vi "ConexionSerial_Clase3.vi"() -> ()   [LabVIEW 2017]
uses:
  <vilib>/Instr/_visa.llb/VISA Configure Serial Port (Instr).vi
panel:
  out "x+/-y":i8
  in  "stop":bool
  out "read buffer":string
  in  "VISA resource name":refnum<visa-resource-name>
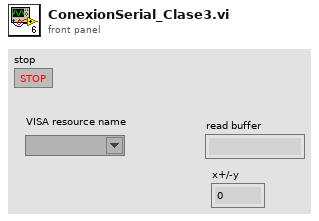
[diagram p1: front panel]
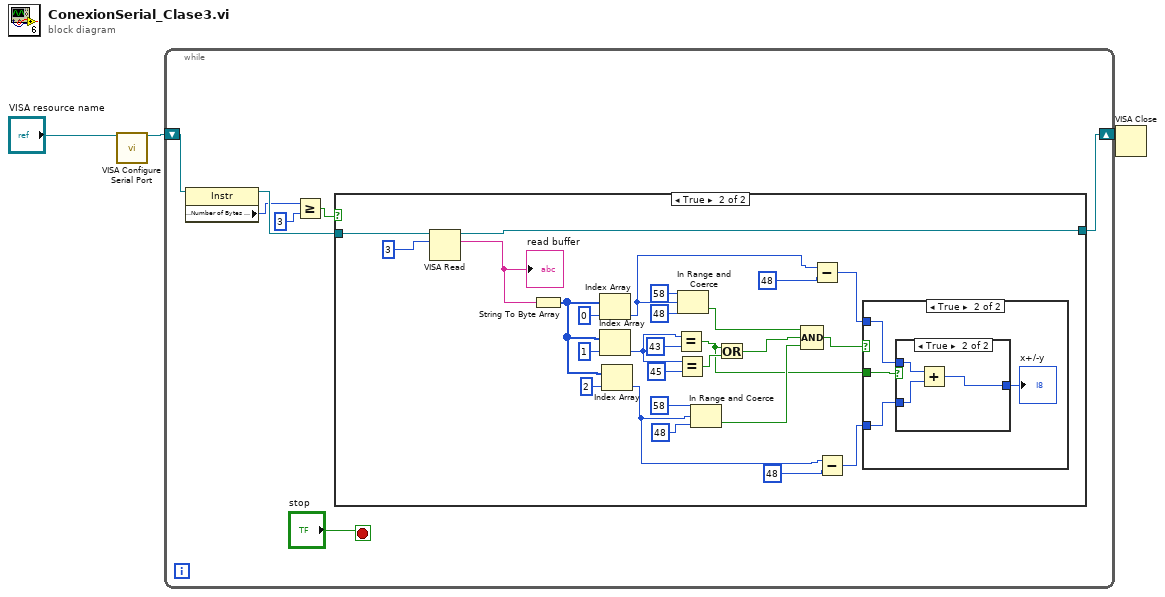
[diagram p0: block diagram]
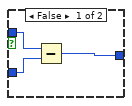
[diagram p4: hidden frame]
diagram:
  n1 = call-poly "VISA Configure Serial Port"("VISA resource name"="VISA resource name") -> ("VISA resource name out"=w2:refnum<visa-resource-name>)  [unwired: 13 in, 1 out]
  n2 = while {
    shift-right: [w10] -> w1
    shift-left: w2 -> [w8]
    stop <- "stop" stop-if-true
    n3 = property class="Instr"(reference=w8) -> (reference out=w7:refnum<visa-resource-name>, "Serial Settings:Number of Bytes at Serial Port"=w4:u32)  [unwired: 1 in, 1 out]
    n4 = Greater Or Equal?(x=w4, y=u32 3 ("x")) -> (x >= y?=w6:bool)
    n5 = case shown="True" w6 {
      tunnel: w7 -> [w11 w38]
      tunnel: [w11 w36] -> w10
      frame False {
      }
      frame True {
        n6 = VISA Read(VISA resource name=w38, byte count=u32 3) -> (VISA resource name out=w36:refnum<visa-resource-name>, read buffer=w35:string)  [unwired: 1 in, 2 out]
        "read buffer" <- w35
        n7 = String To Byte Array(string=w35) -> (unsigned byte array=w31:u8[])
        n8 = Index Array(array=w31, index=0) -> (element=w17:u8)
        n9 = Index Array(array=w31, index=1) -> (element=w26:u8)
        n10 = Index Array(array=w31, index=2) -> (element=w13:u8)
        n11 = Equal?(x=w26, y=u8 43) -> (x = y?=w18:bool)
        n12 = Equal?(x=w26, y=u8 45) -> (x = y?=w23:bool)
        n13 = In Range and Coerce(upper limit=u8 58, x=w17, lower limit=u8 48) -> (In Range?=w22:bool)  [unwired: 1 out]
        n14 = In Range and Coerce(upper limit=u8 58, x=w13, lower limit=u8 48) -> (In Range?=w20:bool)  [unwired: 1 out]
        n15 = Or(x=w18, y=w23) -> (x .or. y?=w21:bool)
        n16 = Compound Arithmetic op=AND(w22, w21, w20) -> (w19:bool)
        n17 = Subtract(x=w17, y=u8 48) -> (x-y=w15:u8)
        n18 = Subtract(x=w13, y=u8 48) -> (x-y=w12:u8)
        n19 = case shown="True" w19 {
          tunnel: w18 -> [_ w42]
          tunnel: w15 -> [_ w41]
          tunnel: w12 -> [_ w40]
          frame False {
          }
          frame True {
            n20 = case shown="True" w42 {
              tunnel: w41 -> [w45 w48]
              tunnel: w40 -> [w44 w47]
              tunnel: [w43 w46] -> w39
              frame False {
                n21 = Subtract(x=w45, y=w44) -> (x-y=w43:u8)
              }
              frame True {
                n22 = Add(x=w48, y=w47) -> (x+y=w46:u8)
              }
            }
            "x+/-y" <- w39
          }
        }
      }
    }
  }
  n23 = VISA Close(VISA resource name=w1) -> ()  [unwired: 1 in, 1 out]
